vi "人數.vi"() -> (0 "三人 3":bool, 1 "4":bool, 2 "3":bool, 3 "2":bool)   [LabVIEW 2014]
panel:
  in  "白色恐怖":bool
  in  "四人":bool
  in  "三人":bool
  in  "雙人":bool
  in  "Color Box":u32(colorbox)=16768479
  # "歡迎來到LabVIEW大富翁"
  # "請選擇遊戲人數"
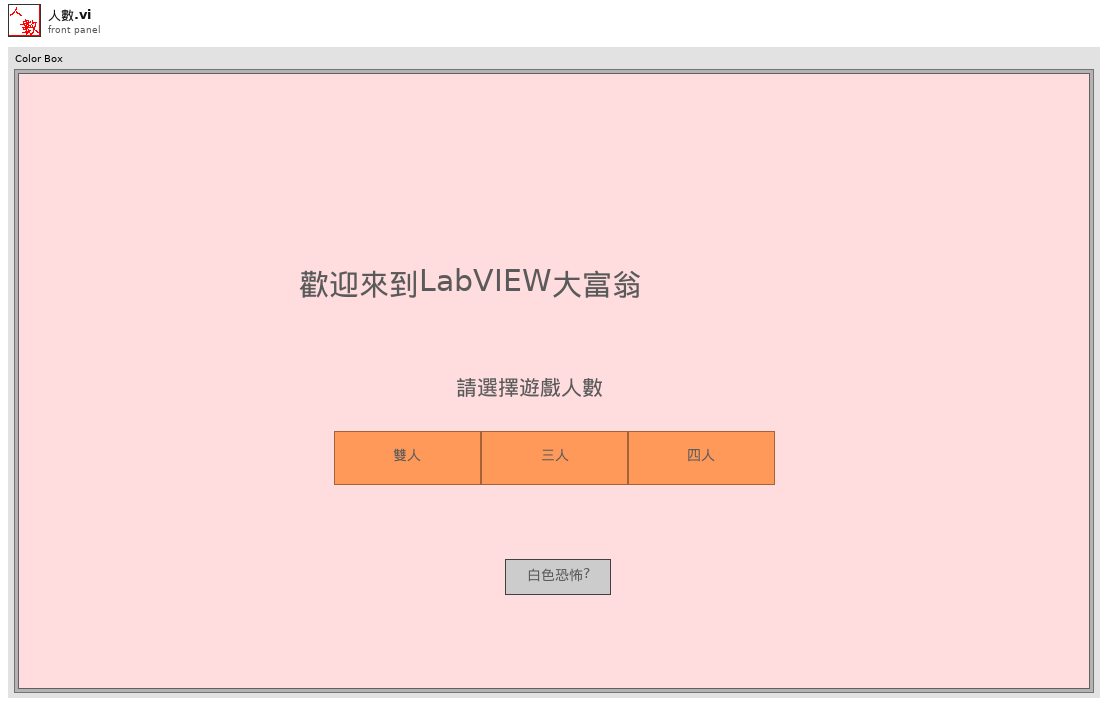
[diagram p1: front panel]
types:
  T1 = enum8{"Enabled", "Disabled", "Disabled and Grayed Out"}
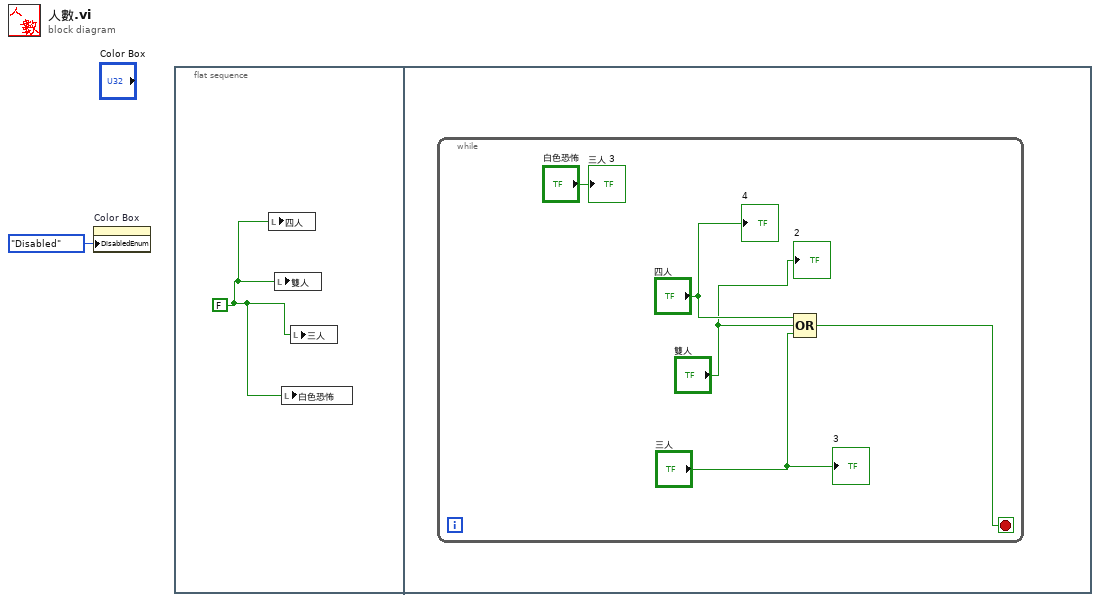
[diagram p0: block diagram]
diagram:
  n1 = property on="Color Box" class="ColBox"("DisabledEnum"=T1."Disabled" ("Disabled")) -> ()  [unwired: 2 in, 2 out]
  n2 = flat-sequence {
    frame #0 {
      w2 = FALSE
      n3 = local write "四人"(w2) -> ()
      n4 = local write "雙人"(w2) -> ()
      n5 = local write "白色恐怖"(w2) -> ()
      n6 = local write "三人"(w2) -> ()
    }
    frame #1 {
      n7 = while {
        stop <- w7 stop-if-true
        n8 = Compound Arithmetic op=OR("四人", "雙人", "三人") -> (w7:bool)
        "2" <- "雙人"
        "3" <- "三人"
        "4" <- "四人"
        "三人 3" <- "白色恐怖"
      }
    }
  }
